vi "Colour_Prediction.vi"() -> ()   [LabVIEW 2017]
doc: "The myRIO Project template acquires acceleration data from the onboard accelerometer and displays the changes of acceleration values in a waveform chart."
panel:
  out "min index(es)":i32
  in  "Stop Button":bool
  out "Distances":dbl[](array[numeric])
  out "subarray w clr classifying numbers - within angle range":dbl[][](array[numeric])
  out "lower limit":dbl
  out "upper limit":dbl
  out "Angle":dbl
  in  "?":tag="B/I2C"
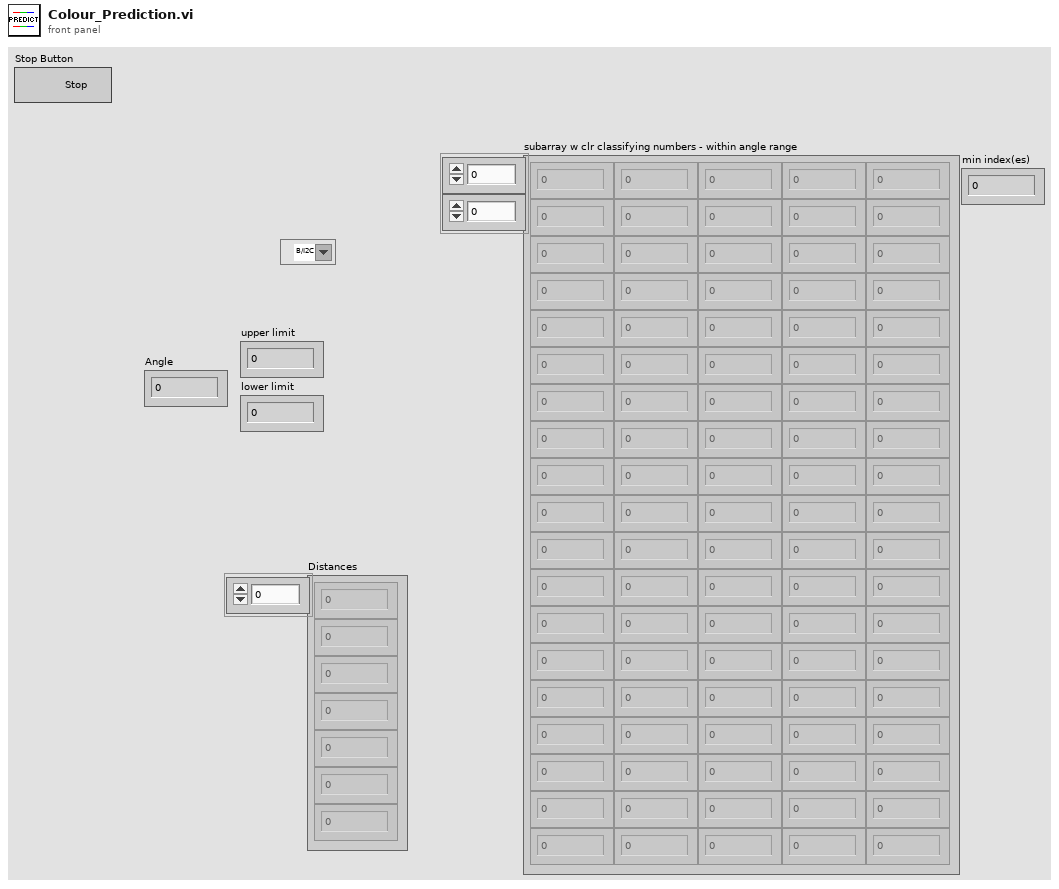
[diagram p1: front panel]
types:
  T1 = typedef "I2C.lvlib/I2C Reference.ctl" = cluster{"myRIO Reference":T2, "I2C Channels Enum":T6, "I2C Configuration":T7}
  T2 = typedef "myRIO Generic Hardware Reference.ctl" = cluster{"myRIO Model":T3, "myRIO Hardware Reference":T4}
  T3 = typedef "Hardware Version Enum.ctl" = enum16{"Unknown", "myRIO-1900", "myRIO-1950", "roboRIO", "NI ELVIS RIO CM"}
  T4 = typedef "myRIO v1.0 Reference.ctl" = cluster{"Generic FPGA Reference":T5, "Allow multiple opens":bool}
  T5 = typedef "Generic FPGA Reference.ctl" = refnum<k20>
  T6 = typedef "I2C Channels Enum.ctl" = enum16{"Not Connected", "A/I2C", "B/I2C", "I2C/I2C"}
  T7 = typedef "I2C.lvlib/I2C Configuration.ctl" = cluster{"I2C Transfer Rate":T8}
  T8 = typedef "I2C.lvlib/I2C Transfer Rate.ctl" = enum16{"Standard mode (100 kbps)", "Fast mode (400 kbps)"}
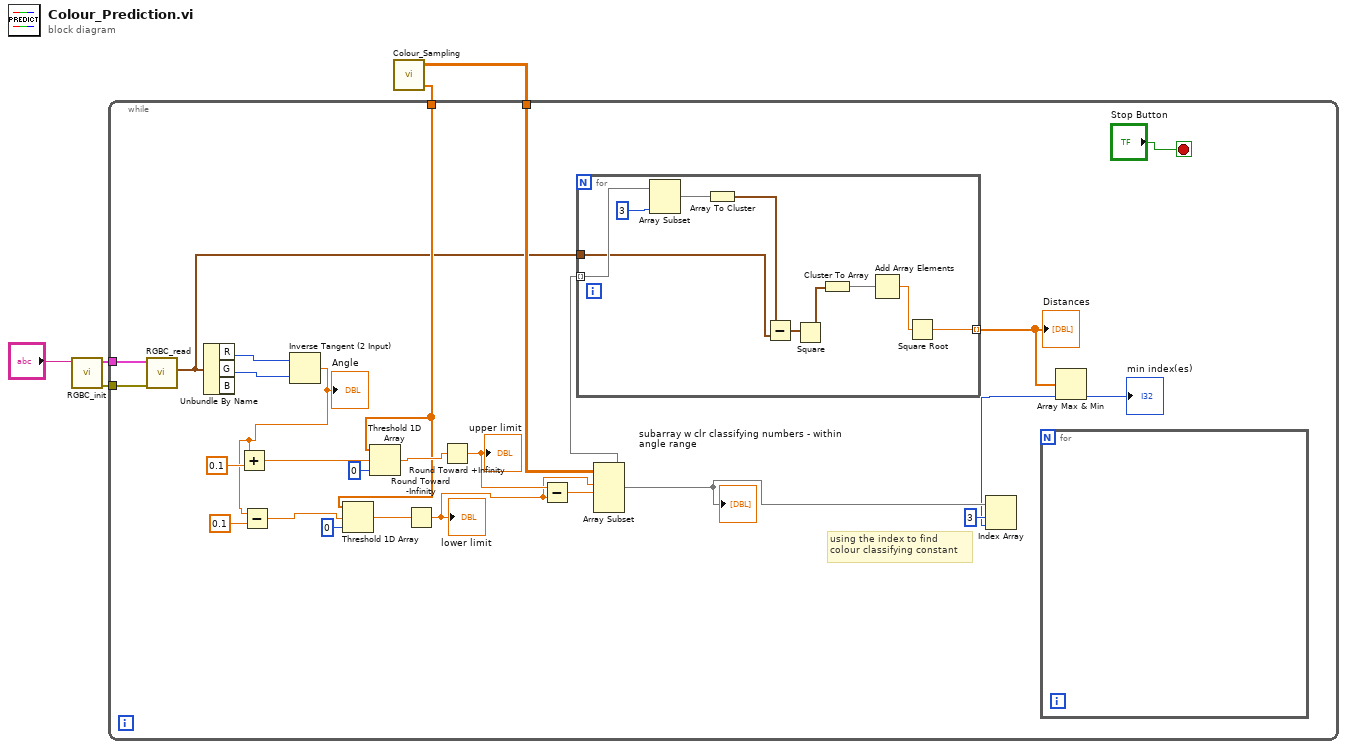
[diagram p0: block diagram]
diagram:
  n1 = call "RGBC_init.vi"("Channel Name"="?") -> ("error out"=w3:errorcluster, "I2C Ref Out"=w4:T1)  [unwired: 9 in]
  n2 = call "Colour_Sampling.vi"() -> ("Just the ascending angles"=w2:dbl[], "All colours in ascending angles: R/G/B/num/angle"=w1:dbl[][])  [unwired: 4 in]
  n3 = while {
    tunnel: w4 -> [w29]
    tunnel: w3 -> [w28]
    tunnel: w2 -> [w12]
    tunnel: w1 -> [w11]
    stop <- "Stop Button" stop-if-true
    # "using the index to find \ncolour classifying constant"
    n4 = call "RGBC_read.vi"("error in (no error)"=w28, "I2C Ref In"=w29) -> ("RGB"=w10:cluster{"R":u8, "G":u8, "B":u8})  [unwired: 7 in, 2 out]
    n5 = Unbundle By Name(w10) -> ("R"=w15:u8, "G"=w14:u8)  [unwired: 1 out]
    n6 = Inverse Tangent (2 Input)(1:w14, 2:w15) -> (0:w24:dbl)
    "Angle" <- w24
    n7 = Add(x=w24, y=0.1) -> (x+y=w26:dbl)
    n8 = Subtract(x=w24, y=0.1) -> (x-y=w23:dbl)
    n9 = Threshold 1D Array(1:0 ("start index (0)"), 2:w23, 3:w12) -> (0:w21:dbl)
    n10 = Threshold 1D Array(1:0 ("start index (0)"), 2:w26, 3:w12) -> (0:w22:dbl)
    n11 = Round Toward -Infinity(1:w21) -> (0:w18:dbl)
    "lower limit" <- w18
    n12 = Round Toward +Infinity(x=w22) -> (ceil(x): smallest int >= x=w20:dbl)
    "upper limit" <- w20
    n13 = Subtract(x=w20, y=w18) -> (x-y=w19:dbl)
    n14 = Array Subset(array=w11, index (row)=w18, length (row)=w19) -> (w9:dbl[][])  [unwired: 2 in]
    "subarray w clr classifying numbers - within angle range" <- w9
    n15 = for {
      tunnel: w9 -> [w37] mode=indexing
      tunnel: [w39] -> w6 mode=indexing
      tunnel: w10 -> [w34]
      n16 = Array Subset(array=w37, length=3) -> (w35:dbl[])  [unwired: 1 in]
      n17 = Array To Cluster(array=w35) -> (cluster=w33:cluster{"[0]":dbl, "[1]":dbl, "[2]":dbl})
      n18 = Subtract(x=w33, y=w34) -> (x-y=w38:cluster{dbl, dbl, dbl})
      n19 = Square(x=w38) -> (x^2=w32:cluster{dbl, dbl, dbl})
      n20 = Cluster To Array(cluster=w32) -> (array=w31:dbl[])
      n21 = Add Array Elements(numeric array=w31) -> (sum=w30:dbl)
      n22 = Square Root(x=w30) -> (sqrt(x)=w39:dbl)
    }
    "Distances" <- w6
    n23 = for {
    }
    n24 = Array Max & Min(array=w6) -> (min index (indices)=w7:i32)  [unwired: 3 out]
    "min index(es)" <- w7
    n25 = Index Array(array=w9, index (row)=3, index (col)=w7) -> ()  [unwired: 1 out]
  }
